vi "Remove String Spaces.vi"(8 "error in (no error)":errorcluster, 11 "Input String":string) -> (0 "error out":errorcluster, 2 "Output String":string)   [LabVIEW 2016, in "Assert API Components.lvlib" / "Assert Startup UI.lvlib" / "Assert Startup UI.lvclass"]
uses:
  Assert Startup UI.lvclass
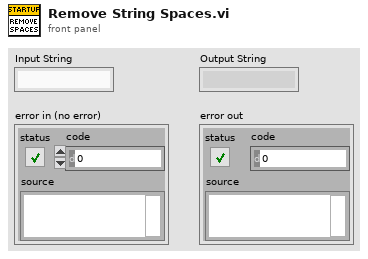
[diagram p1: front panel]
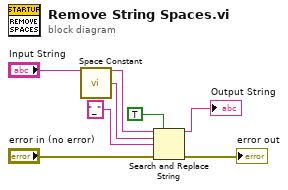
[diagram p0: block diagram]
diagram:
  n1 = call <vilib>:"Space Constant.vi"() -> ("String"=w4:string)
  n2 = Search and Replace String(replace all?=TRUE ("replace all? (F)"), input string="Input String", search string=w4, replace string="_" ("replace string (\"\")"), error in="error in (no error)") -> (result string=→"Output String":string, error out=→"error out":errorcluster)  [unwired: 3 in, 2 out]
